vi "SRV_Update Status Indicator.vi"(0 "Status ref":refnum<vi>, 5 "Status":string, 11 "error in (no error)":errorcluster, 12 "Delay After Update (0 ms)":u32) -> (4 "Status ref out":refnum<vi>, 15 "error out":errorcluster)   [LabVIEW 2014]
doc: "Update the value property of the string referenced by \"Status ref\".\n\n\nAuthor: Mike Schultz - Logic PD"
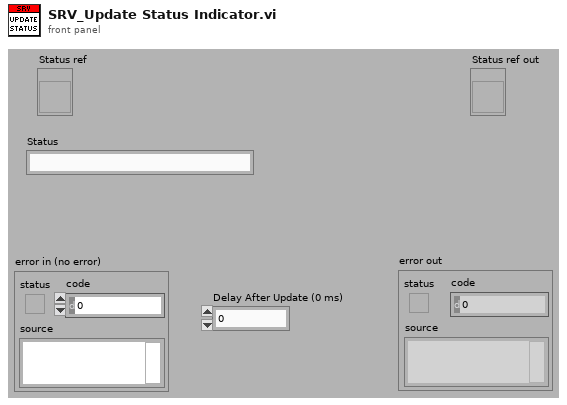
[diagram p1: front panel]
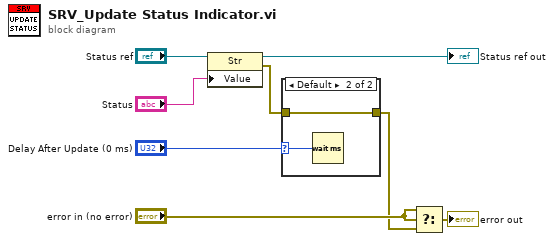
[diagram p0: block diagram]
diagram:
  n1 = property class="Str"(reference="Status ref", "Value"="Status") -> (reference out=→"Status ref out":refnum<vi>, error out=w4:errorcluster)  [unwired: 1 in]
  n2 = case shown="Default" "Delay After Update (0 ms)" {
    selector: "Delay After Update (0 ms)" -> [_ w11]
    tunnel: w4 -> [w9 w10]
    tunnel: [w9 w10] -> w1
    frame 0 {
    }
    frame Default {
      n3 = Wait (ms)(milliseconds to wait=w11) -> ()  [unwired: 1 out]
    }
  }
  n4 = Select(t="error in (no error)", s="error in (no error)", f=w1) -> (s? t:f=→"error out":errorcluster)
